vi "Read TV DisplayCtr Color.vi"(8 "error in (no error)":errorcluster, 11 "Path":path) -> (0 "error out":errorcluster, 1 "Color":T2, 2 "Range":T1, 3 "Array":cluster{"Label":string, "Color":u32}[](array[cluster]))   [LabVIEW 2014]
uses:
  <vilib>/Utility/config.llb/Read Key (U32).vi
  <vilib>/Utility/config.llb/NI_LVConfig.lvlib
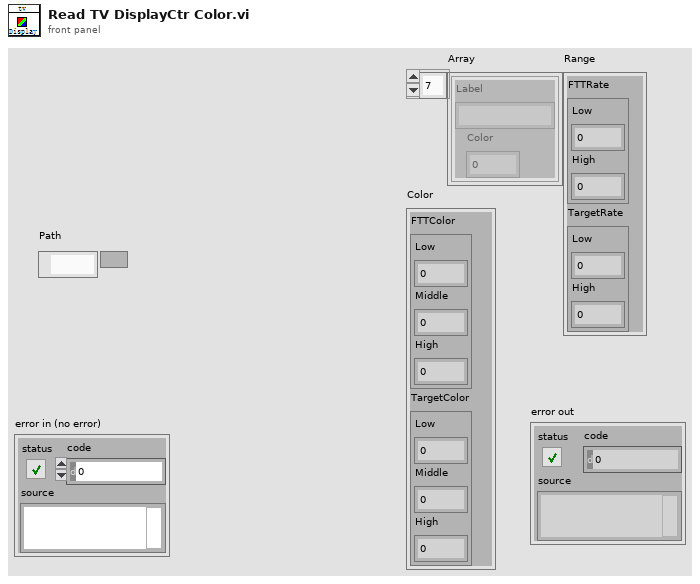
[diagram p1: front panel]
types:
  T1 = cluster{"FTTRate":cluster{"Low":u32, "High":u32}, "TargetRate":cluster{"Low":u32, "High":u32}}
  T2 = cluster{"FTTColor":cluster{"Low":u32, "Middle":u32, "High":u32}, "TargetColor":cluster{"Low":u32, "Middle":u32, "High":u32}}
  T3 = typedef "NI_LVConfig.lvlib/Config Data RefNum.ctl" = refnum<k1>
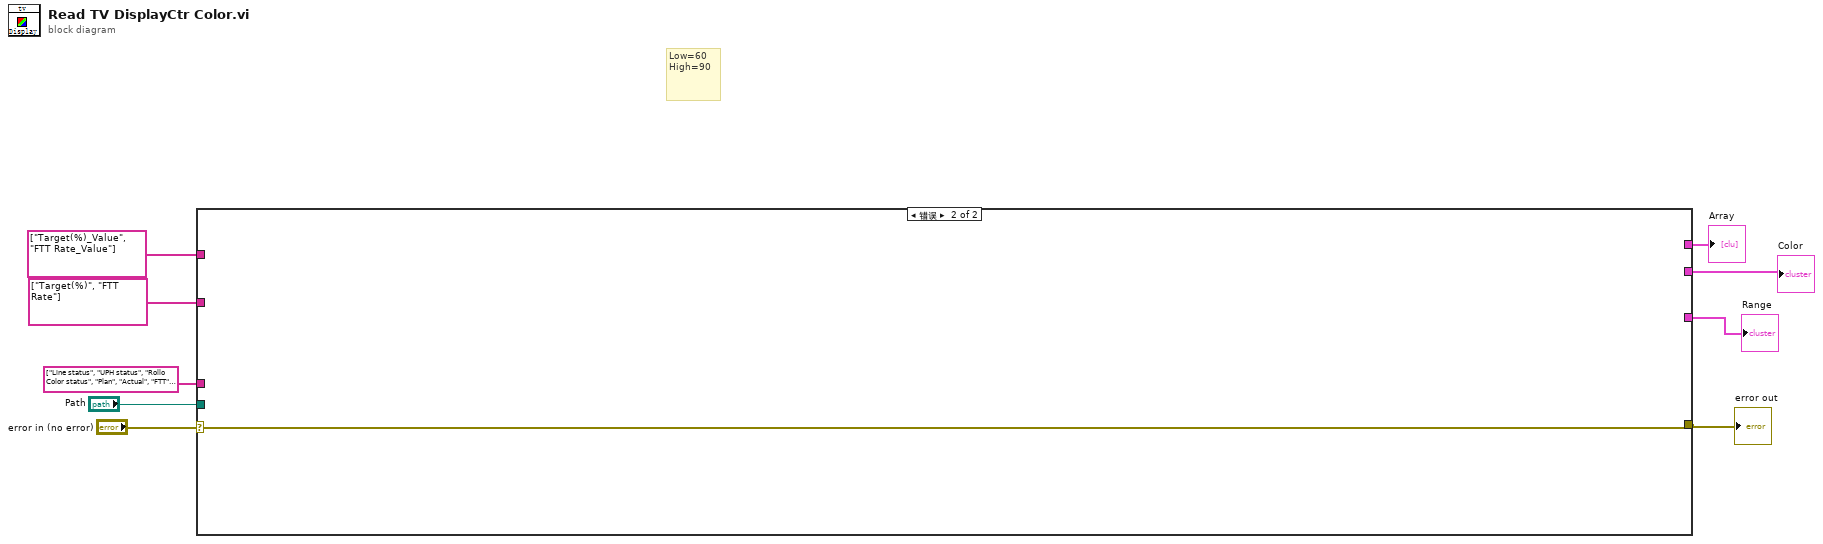
[diagram p0: block diagram]
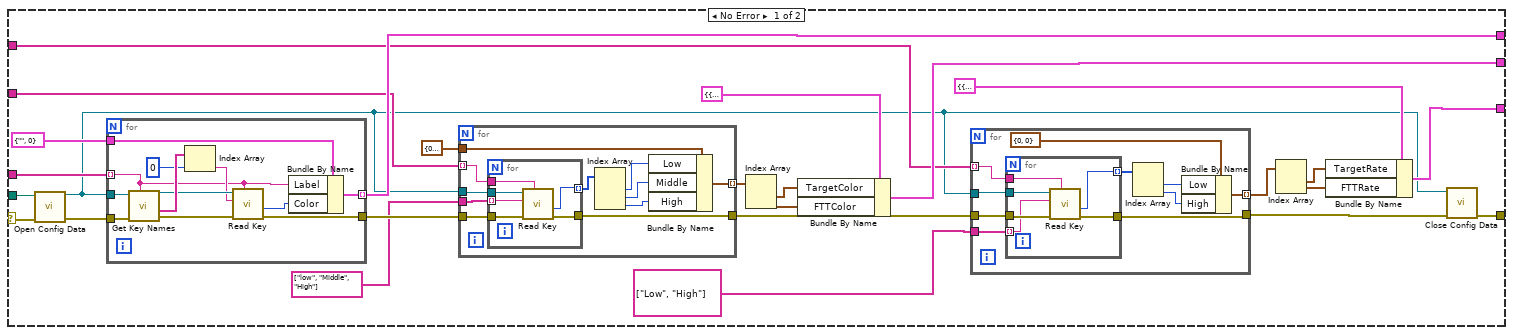
[diagram p2: hidden frame]
diagram:
  # "Low=60\nHigh=90"
  n1 = case shown="错误" "error in (no error)" {
    selector: "error in (no error)" -> [w35 w81]
    tunnel: "Path" -> [w34 _]
    tunnel: string[] ["Line status", "UPH status", "Rollo Color status", "Plan", "Actual", "FTT", "Repaired", "Target now", "Reject"] ("Array") -> [w32 _]
    tunnel: [w30 _] -> w6
    tunnel: string[] ["Target(%)_Value", "FTT Rate_Value"] -> [w18 _]
    tunnel: string[] ["Target(%)", "FTT Rate"] -> [w28 _]
    tunnel: [w21 _] -> w2
    tunnel: [w13 _] -> w1
    tunnel: [w10 w81] -> w3
    frame No Error {
      n2 = call <vilib>:"Open Config Data.vi"("error in (no error)"=w35, "configuration file path"=w34) -> ("error out"=w33:errorcluster, "refnum"=w11:T3)  [unwired: 7 in, 1 out]
      n3 = for {
        tunnel: w33 -> [w80]
        tunnel: w11 -> [w79]
        tunnel: w32 -> [w70] mode=indexing
        tunnel: cluster{"Label":string, "Color":u32} {"Label"="", "Color"=0} ("Ctr Color") -> [w73]
        tunnel: [w71] -> w30 mode=indexing
        tunnel: [w69] -> w29
        n4 = call <vilib>:"Get Key Names.vi"("section"=w70, "error in (no error)"=w80, "refnum"=w79) -> ("error out"=w76:errorcluster, "key names"=w78:string[], "refnum out"=w75:T3)  [unwired: 5 in, 1 out]
        n5 = Index Array(array=w78, index=0) -> (element=w74:string)
        n6 = call-poly <vilib>:"Read Key.vi"("section"=w70, "error in (no error)"=w76, "key"=w74, "refnum"=w75) -> ("error out"=w69:errorcluster, "value"=w72:u32)  [unwired: 4 in, 2 out]
        n7 = Bundle By Name(cluster=w73, "Label"=w70, "Color"=w72) -> (w71:cluster{"Label":string, "Color":u32})
      }
      n8 = for {
        tunnel: w11 -> [w62]
        tunnel: w29 -> [w61]
        tunnel: w28 -> [w60] mode=indexing
        tunnel: string[] ["low", "Middle", "High"] ("Array") -> [w59]
        tunnel: cluster{"Low":u32, "Middle":u32, "High":u32} {"Low"=0, "Middle"=0, "High"=0} ("FTTColor") -> [w57]
        tunnel: [w58] -> w20
        tunnel: [w52] -> w25 mode=indexing
        n9 = for {
          tunnel: w62 -> [w68]
          tunnel: w61 -> [w67]
          tunnel: w60 -> [w66]
          tunnel: w59 -> [w65] mode=indexing
          tunnel: [w64] -> w58
          tunnel: [w63] -> w56 mode=indexing
          n10 = call-poly <vilib>:"Read Key.vi"("section"=w66, "error in (no error)"=w67, "key"=w65, "refnum"=w68) -> ("error out"=w64:errorcluster, "value"=w63:u32)  [unwired: 4 in, 2 out]
        }
        n11 = Index Array(array=w56) -> (element #1=w55:u32, element #2=w54:u32, element #3=w53:u32)  [unwired: 3 in]
        n12 = Bundle By Name(cluster=w57, "Low"=w55, "Middle"=w54, "High"=w53) -> (w52:cluster{"Low":u32, "Middle":u32, "High":u32})
      }
      n13 = Index Array(array=w25) -> (element #1=w23:cluster{"Low":u32, "Middle":u32, "High":u32}, element #2=w22:cluster{"Low":u32, "Middle":u32, "High":u32})  [unwired: 2 in]
      n14 = Bundle By Name(cluster=T2 {"FTTColor"={"Low"=0, "Middle"=0, "High"=0}, "TargetColor"={"Low"=0, "Middle"=0, "High"=0}} ("Color"), "TargetColor"=w23, "FTTColor"=w22) -> (w21:T2)
      n15 = for {
        tunnel: w20 -> [w45]
        tunnel: w11 -> [w44]
        tunnel: string[] ["Low", "High"] -> [w42]
        tunnel: w18 -> [w43] mode=indexing
        tunnel: [w37] -> w17 mode=indexing
        tunnel: [w36] -> w12
        n16 = for {
          tunnel: w45 -> [w51]
          tunnel: w44 -> [w50]
          tunnel: w43 -> [w49]
          tunnel: w42 -> [w48] mode=indexing
          tunnel: [w47] -> w36
          tunnel: [w46] -> w41 mode=indexing
          n17 = call-poly <vilib>:"Read Key.vi"("section"=w49, "error in (no error)"=w51, "key"=w48, "refnum"=w50) -> ("error out"=w47:errorcluster, "value"=w46:u32)  [unwired: 4 in, 2 out]
        }
        n18 = Index Array(array=w41) -> (element #1=w39:u32, element #2=w38:u32)  [unwired: 2 in]
        n19 = Bundle By Name(cluster=cluster{"Low":u32, "High":u32} {"Low"=0, "High"=0} ("FTTRate"), "Low"=w39, "High"=w38) -> (w37:cluster{"Low":u32, "High":u32})
      }
      n20 = Index Array(array=w17) -> (element #1=w15:cluster{"Low":u32, "High":u32}, element #2=w14:cluster{"Low":u32, "High":u32})  [unwired: 2 in]
      n21 = Bundle By Name(cluster=T1 {"FTTRate"={"Low"=0, "High"=0}, "TargetRate"={"Low"=0, "High"=0}} ("Range"), "TargetRate"=w15, "FTTRate"=w14) -> (w13:T1)
      n22 = call <vilib>:"Close Config Data.vi"("error in (no error)"=w12, "refnum"=w11) -> ("error out"=w10:errorcluster)  [unwired: 8 in, 1 out]
    }
    frame Error {
    }
  }
  "error out" <- w3
  "Array" <- w6
  "Color" <- w2
  "Range" <- w1
